vi "Send command to printer.vi"(8 "error in (no error)":errorcluster) -> (0 "error out":errorcluster, 1 "return code":i32, 2 "standard error":string, 3 "standard output":string)   [LabVIEW 2023]
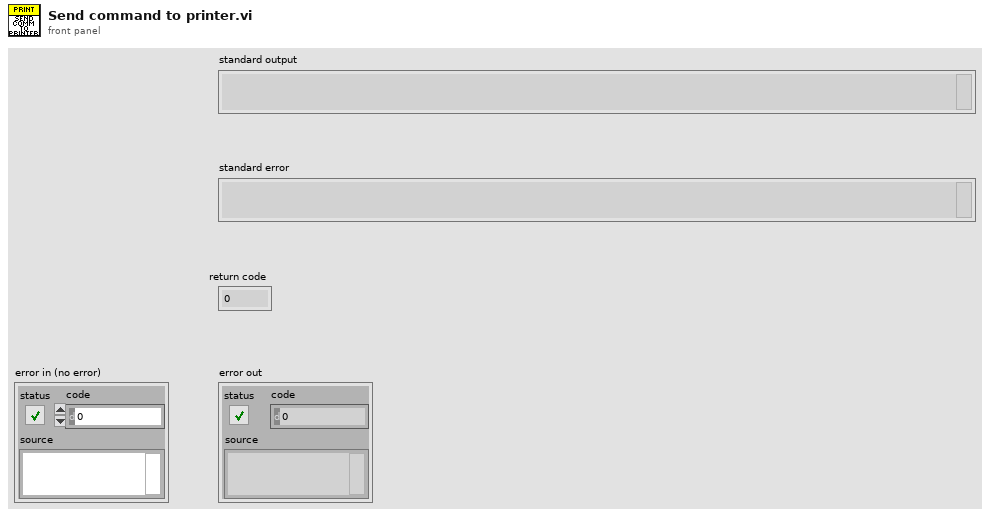
[diagram p1: front panel]
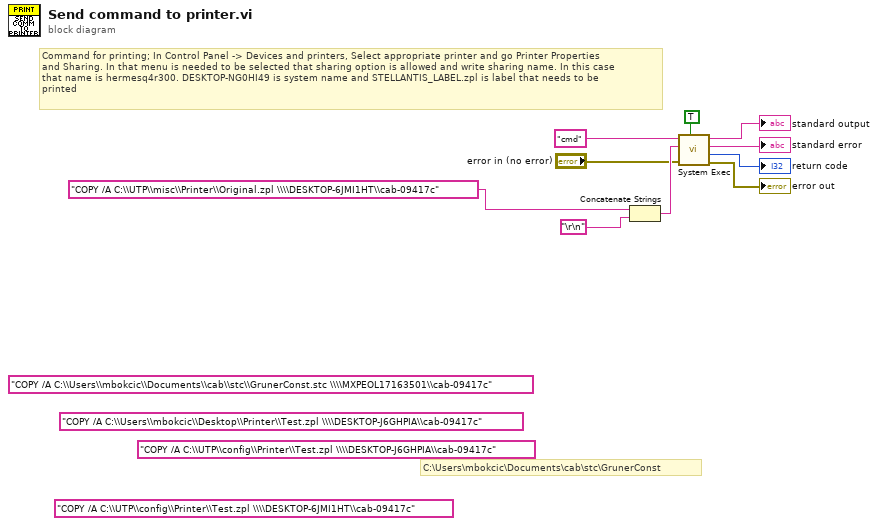
[diagram p0: block diagram]
diagram:
  (unwired) "COPY /A C:\\UTP\\config\\Printer\\Test.zpl \\\\DESKTOP-6JMI1HT\\cab-09417c" ("Print command")
  (unwired) "COPY /A C:\\UTP\\config\\Printer\\Test.zpl \\\\DESKTOP-J6GHPIA\\cab-09417c" ("Print command")
  (unwired) "COPY /A C:\\Users\\mbokcic\\Desktop\\Printer\\Test.zpl \\\\DESKTOP-J6GHPIA\\cab-09417c" ("Print command")
  (unwired) "COPY /A C:\\Users\\mbokcic\\Documents\\cab\\stc\\GrunerConst.stc \\\\MXPEOL17163501\\cab-09417c" ("Print command")
  # "C:\\Users\\mbokcic\\Documents\\cab\\stc\\GrunerConst"
  # "Command for printing; In Control Panel -> Devices and printers, Select appropriate printer and go Printer Properties\nand Sharing. In that menu is needed to be selected that sharing option is allowed and write sharing name. In this case \nthat name is hermesq4r300. DESKTOP-NG0HI49 is system name and STELLANTIS_LABEL.zpl is label that needs to be\nprinted"
  n1 = Concatenate Strings("COPY /A C:\\UTP\\misc\\Printer\\Original.zpl \\\\DESKTOP-6JMI1HT\\cab-09417c" ("Print command"), "\r\n") -> (w7:string)
  n2 = call <vilib>:"System Exec.vi"("wait until completion? (T)"=TRUE, "error in (no error)"="error in (no error)", "standard input"=w7, "command line"="cmd") -> ("error out"=→"error out":errorcluster, "return code"=→"return code":i32, "standard error"=→"standard error":string, "standard output"=→"standard output":string)  [unwired: 4 in]
